vi "Configure Power Sensor Measurement Timeout.vi"(8 "error in (no error)":errorcluster, 9 "Timeout (1)":i32=1, 10 "Instance (1)":i32=1, 11 "VISA resource name":refnum<visa-resource-name>) -> (0 "error out":errorcluster, 3 "VISA resource name out":refnum<visa-resource-name>)   [LabVIEW 2015, in "Rohde&Schwarz CMXP GPRF.lvlib"]
doc: "Defines a timeout for the measurement.\n\nAttribute:\nRSCMXPGPRF_ATTR_POWER_SENSOR_MEASUREMENT_TIMEOUT\n\nRemote-control command:\nCONFigure:GPRF:MEAS<i>:EPSensor:TOUT"
uses:
  <instrlib>/Rohde&Schwarz CMXP GPRF/Rohde&Schwarz CMXP GPRF.lvlib
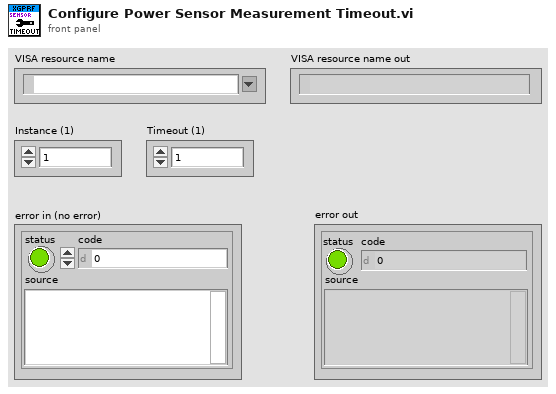
[diagram p1: front panel]
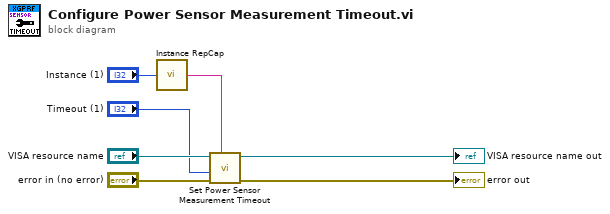
[diagram p0: block diagram]
diagram:
  n1 = call <instrlib>:"Instance RepCap.vi"("instance  in"="Instance (1)") -> ("instance out"=w6:string)
  n2 = call "Set Power Sensor Measurement Timeout"("Repeated Capabilities"=w6, "error in (no error)"="error in (no error)", "Power Sensor Measurement Timeout (0.0)"="Timeout (1)", "instrument handle"="VISA resource name") -> ("error out"=→"error out":errorcluster, "instrument handle out"=→"VISA resource name out":refnum<visa-resource-name>)  [unwired: 6 in]
